vi "Escape Percents.vi"(4 "String in":string) -> (7 "String":string)   [LabVIEW 2020, in "VolatusGUIEditorCore.lvlib"]
uses:
  VolatusGUIEditorCore.lvlib
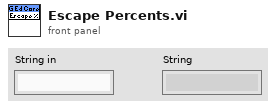
[diagram p1: front panel]
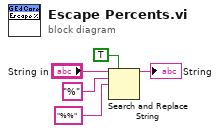
[diagram p0: block diagram]
diagram:
  n1 = Search and Replace String(replace all?=TRUE ("replace all? (F)"), input string="String in", search string="%", replace string="%%" ("search string")) -> (result string=→"String":string)  [unwired: 4 in, 3 out]
